vi "20170411-lecture3-global variable2.vi"() -> ()   [LabVIEW 2014]
uses:
  20170411-lecture3-global variable.vi
panel:
  out "Chart 1":dbl(graph)
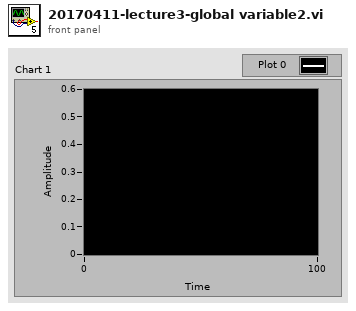
[diagram p1: front panel]
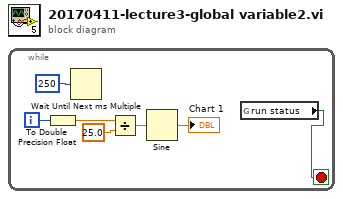
[diagram p0: block diagram]
diagram:
  n1 = while {
    i -> [w2]
    stop <- w1 stop-if-true
    n2 = To Double Precision Float(number=w2) -> (double precision float=w3:dbl)
    n3 = Wait Until Next ms Multiple(millisecond multiple=u32 250) -> ()  [unwired: 1 out]
    n4 = Divide(x=w3, y=25.0) -> (x/y=w7:dbl)
    n5 = Sine(x=w7) -> (sin(x)=→"Chart 1":dbl)
    n6 = global read "20170411-lecture3-global variable.vi" "run status"() -> (w1:bool)
  }
